vi "ROS_ParseMsgFile.vi"() -> ()   [LabVIEW 2012]
panel:
  in  "msg file":string
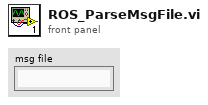
[diagram p1: front panel]
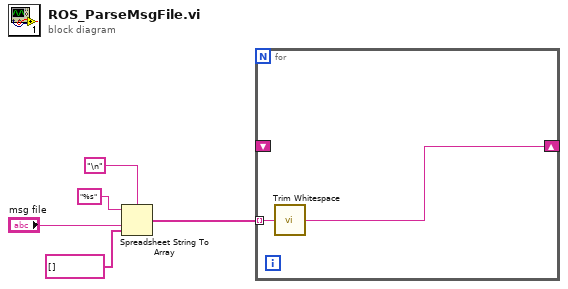
[diagram p0: block diagram]
diagram:
  n1 = Spreadsheet String To Array(delimiter (Tab)="\n", format string="%s", spreadsheet string="msg file", array type (2D Dbl)=string[] []) -> (array=w1:string[])
  n2 = for {
    tunnel: w1 -> [w7] mode=indexing
    shift-right: [w6] -> _
    shift-left: _ -> [_]
    n3 = call <vilib>:"Trim Whitespace.vi"("string"=w7) -> ("trimmed string"=w6:string)  [unwired: 1 in]
  }
